vi "Factory reset.vi"(8 "error in (no error)":errorcluster, 11 "JSONRead in":T1) -> (0 "error out":errorcluster)   [LabVIEW 2019, in "ZenGage v3.0 UI.lvclass"]
uses:
  ZenGage v3.0 UI.lvclass
  User Interface Messages/User Interface messages/Display Popup Msg/DisplayPopup_UI.lvclass
  Common/Controls/Pop-up Input.ctl
  <vilib>/ActorFramework/Message Enqueuer/Message Enqueuer.lvclass
  Type Definitions/JSON Read/UI JSON read cluster.ctl
  Type Definitions/General/JSONRead.ctl
panel:
  in  "parts List":string[](array[string])
  in  "UI enqueuer":refnum<class "Message Enqueuer.lvclass">
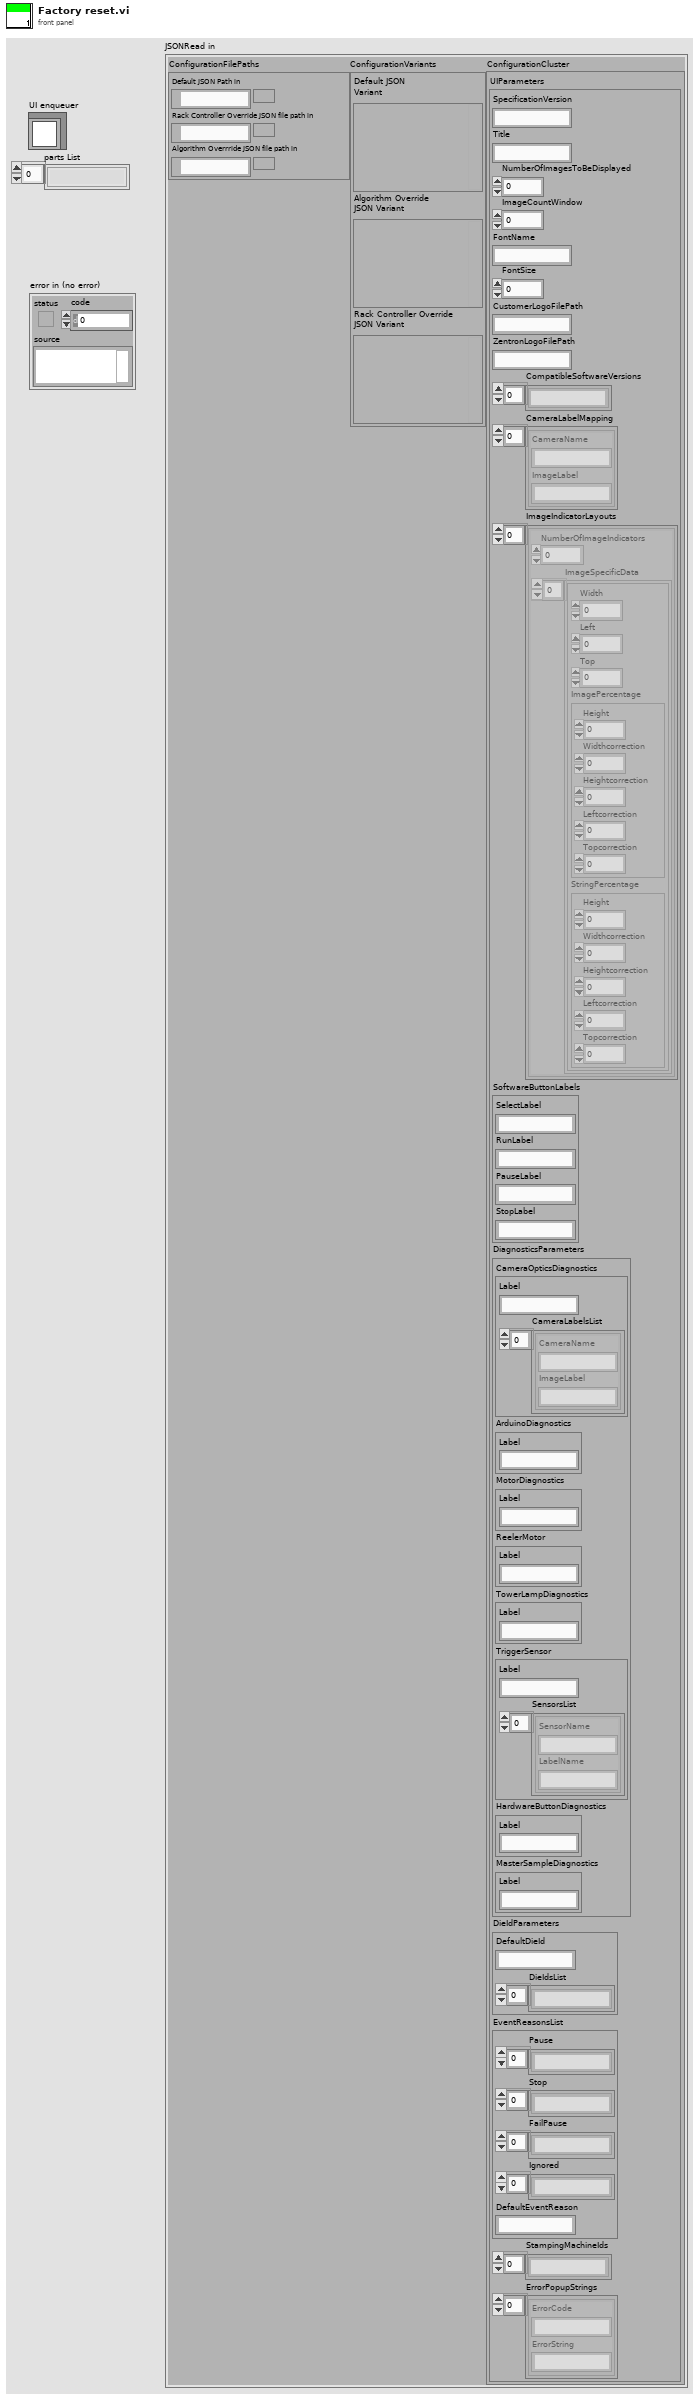
[diagram p1: front panel]
types:
  T1 = typedef "ZenGage v3.0 UI.lvclass/JSONRead.ctl" = cluster{"ConfigurationFilePaths":cluster{"Default JSON Path in":path, "Rack Controller Override JSON file path in":path, "Algorithm Overrride JSON file path in ":path}, "ConfigurationVariants":cluster{"Default JSON \nVariant":variant, "Algorithm Override\nJSON Variant":variant, "Rack Controller Override\nJSON Variant":variant}, "ConfigurationCluster":T2}
  T2 = typedef "ZenGage v3.0 UI.lvclass/UI JSON read cluster.ctl" = cluster{"UIParameters":cluster{"SpecificationVersion":string, "Title":string, "NumberOfImagesToBeDisplayed":dbl, "ImageCountWindow":dbl, "FontName":string, "FontSize":dbl, "CustomerLogoFilePath":string, "ZentronLogoFilePath":string, "CompatibleSoftwareVersions":string[], "CameraLabelMapping":cluster{"CameraName":string, "ImageLabel":string}[], "ImageIndicatorLayouts":cluster{"NumberOfImageIndicators":dbl, "ImageSpecificData":cluster{"Width":dbl, "Left":dbl, "Top":dbl, "ImagePercentage":cluster{"Height":dbl, "Widthcorrection":i64, "Heightcorrection":i64, "Leftcorrection":dbl, "Topcorrection":dbl}, "StringPercentage":cluster{"Height":dbl, "Widthcorrection":i64, "Heightcorrection":dbl, "Leftcorrection":dbl, "Topcorrection":dbl}}[]}[], "SoftwareButtonLabels":cluster{"SelectLabel":string, "RunLabel":string, "PauseLabel":string, "StopLabel":string}, "DiagnosticsParameters":cluster{"CameraOpticsDiagnostics":cluster{"Label":string, "CameraLabelsList":cluster{"CameraName":string, "ImageLabel":string}[]}, "ArduinoDiagnostics":cluster{"Label":string}, "MotorDiagnostics":cluster{"Label":string}, "ReelerMotor":cluster{"Label":string}, "TowerLampDiagnostics":cluster{"Label":string}, "TriggerSensor":cluster{"Label":string, "SensorsList":cluster{"SensorName":string, "LabelName":string}[]}, "HardwareButtonDiagnostics":cluster{"Label":string}, "MasterSampleDiagnostics":cluster{"Label":string}}, "DieIdParameters":cluster{"DefaultDieId":string, "DieIdsList":string[]}, "EventReasonsList":cluster{"Pause":string[], "Stop":string[], "FailPause":string[], "Ignored":string[], "DefaultEventReason":string}, "StampingMachineIds":string[], "ErrorPopupStrings":cluster{"ErrorCode":string, "ErrorString":string}[]}}
  T3 = enum16{"Open Logo Display", "Close Logo Display", "Open Loading Bar", "Close Loading Bar", "Open Alert Display", "Close Alert Display", "One button dialog box", "Two button dialog box", "User Authentication"}
  T4 = typedef "Pop-up Input.ctl" = cluster{"Pop-up Type":enum16{"Open Logo Display", "Close Logo Display", "Open Loading Bar", "Close Loading Bar", "Open Alert Display", "Close Alert Display", "One button dialog box", "Two button dialog box", "User Authentication"}, "Title":string, "Message":string, "Button 1 Text":string, "Button 2 Text":string, "Show Close? T/F":bool, "Title Blink? T/F":bool, "Title Blink Colour":u32}
  T5 = cluster{"Default JSON file path in":path, "Rack Controller Override JSON file path in":path, "Algo Parameters Override JSON file path in":path}
  T6 = cluster{"Default Override JSON":variant, "Rack Controller Override JSON":variant, "Algo Override JSON":variant}
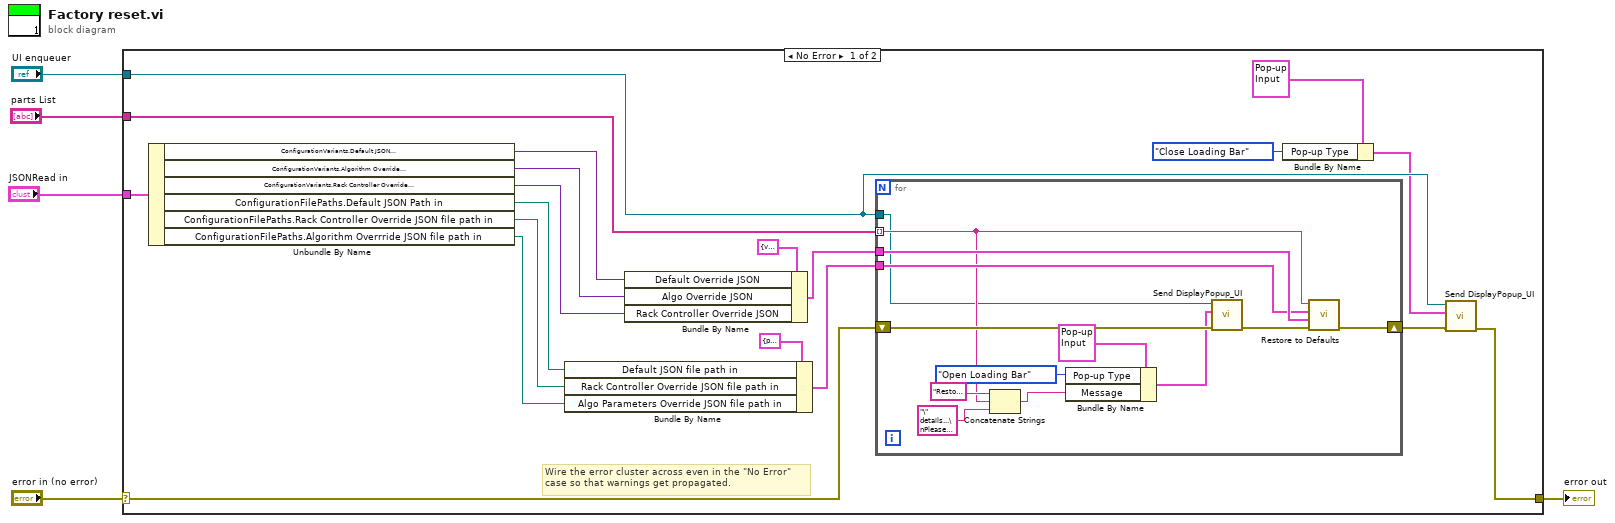
[diagram p0: block diagram]
diagram:
  n1 = case shown="No Error" "error in (no error)" {
    selector: "error in (no error)" -> [w13 w38]
    tunnel: [w11 w38] -> w4
    tunnel: "JSONRead in" -> [w22 _]
    tunnel: "UI enqueuer" -> [w10 _]
    tunnel: "parts List" -> [w6 _]
    frame No Error {
      # "Wire the error cluster across even in the \"No Error\"\ncase so that warnings get propagated."
      n2 = Unbundle By Name(w22) -> ("ConfigurationVariants.Default JSON \nVariant"=w21:variant, "ConfigurationVariants.Algorithm Override\nJSON Variant"=w20:variant, "ConfigurationVariants.Rack Controller Override\nJSON Variant"=w19:variant, "ConfigurationFilePaths.Default JSON Path in"=w18:path, "ConfigurationFilePaths.Rack Controller Override JSON file path in"=w17:path, "ConfigurationFilePaths.Algorithm Overrride JSON file path in"=w16:path)
      n3 = Bundle By Name(cluster=T5 {"Default JSON file path in"=path "", "Rack Controller Override JSON file path in"=path "", "Algo Parameters Override JSON file path in"=path ""} ("JSON path cluster"), "Default JSON file path in"=w18, "Rack Controller Override JSON file path in"=w17, "Algo Parameters Override JSON file path in"=w16) -> (w14:T5)
      n4 = Bundle By Name(cluster=T6 {"Default Override JSON"=variant, "Rack Controller Override JSON"=variant, "Algo Override JSON"=variant} ("JSON Variant Clusters"), "Default Override JSON"=w21, "Algo Override JSON"=w20, "Rack Controller Override JSON"=w19) -> (w15:T6)
      n5 = for {
        tunnel: w15 -> [w37]
        tunnel: w14 -> [w36]
        tunnel: w6 -> [w32] mode=indexing
        shift-right: [w28] -> w12
        shift-left: w13 -> [w35]
        tunnel: w10 -> [w29]
        n6 = Concatenate Strings("Restoring part \"" ("Loading string?"), w32, "\" details...\nPlease wait..." ("Loading string?")) -> (w30:string)
        n7 = Bundle By Name(cluster=T4 {"Pop-up Type"=enum."Open Logo Display", "Title"="", "Message"="", "Button 1 Text"="", "Button 2 Text"="", "Show Close? T/F"=FALSE, "Title Blink? T/F"=FALSE, "Title Blink Colour"=0} ("PopupDetails"), "Pop-up Type"=T3."Open Loading Bar", "Message"=w30) -> (w25:T4)
        n8 = call "Send DisplayPopup_UI.vi"("error in (no error)"=w35, "PopupDetails"=w25, "Message Enqueuer"=w29) -> ("error out"=w34:errorcluster)  [unwired: 7 in, 1 out]
        n9 = call "Restore to Defaults.vi"("error in"=w34, "JSON Variant Clusters"=w37, "JSON path cluster"=w36, "Part Name in"=w32) -> ("error out"=w28:errorcluster)  [unwired: 5 in, 2 out]
      }
      n10 = Bundle By Name(cluster=T4 {"Pop-up Type"=enum."Open Logo Display", "Title"="", "Message"="", "Button 1 Text"="", "Button 2 Text"="", "Show Close? T/F"=FALSE, "Title Blink? T/F"=FALSE, "Title Blink Colour"=0} ("PopupDetails"), "Pop-up Type"=T3."Close Loading Bar") -> (w8:T4)
      n11 = call "Send DisplayPopup_UI.vi"("error in (no error)"=w12, "PopupDetails"=w8, "Message Enqueuer"=w10) -> ("error out"=w11:errorcluster)  [unwired: 7 in, 1 out]
    }
    frame Error {
    }
  }
  "error out" <- w4
